vi "SalvarConfig.vi"(0 "caminho in":path, 1 "CanaisDinamicos":T2[](array[typedef]), 2 "CanaisEstaticos":string[][](array[string]), 3 "ConfigSistema":T1, 5 "error in":errorcluster) -> (14 "caminho out":path, 19 "error out":errorcluster)   [LabVIEW 2017]
uses:
  Typedefs/Tipo_DadosCanal.ctl
  Typedefs/Tipo_TipoSinalSimulado.ctl
  Typedefs/Tipo_ConfigSistema.ctl
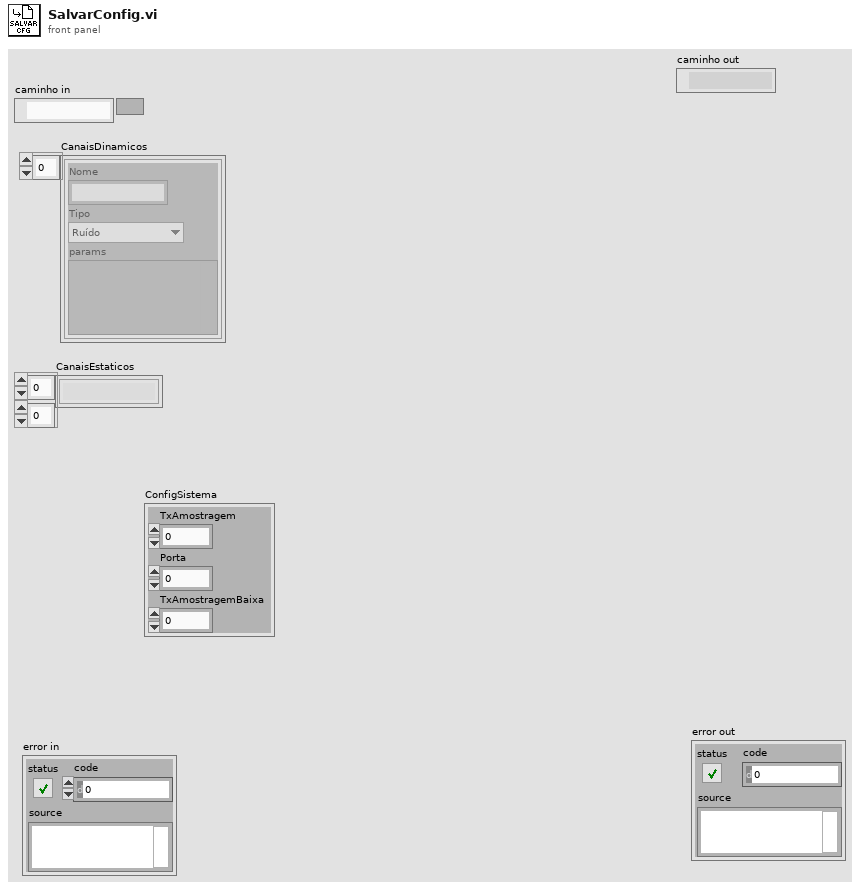
[diagram p1: front panel]
types:
  T1 = typedef "Tipo_ConfigSistema.ctl" = cluster{"TxAmostragem":dbl, "Porta":u16, "TxAmostragemBaixa":dbl}
  T2 = typedef "Tipo_DadosCanal.ctl" = cluster{"Nome":string, "Tipo":T3, "params":variant}
  T3 = typedef "Tipo_TipoSinalSimulado.ctl" = enum16{"Ruído", "Fasor", "Senóide", "Composto", "AM", "Proximidade", "Entreferro"}
  T4 = enum16{"open", "replace", "create", "open or create", "replace or create", "replace or create with confirmation"}
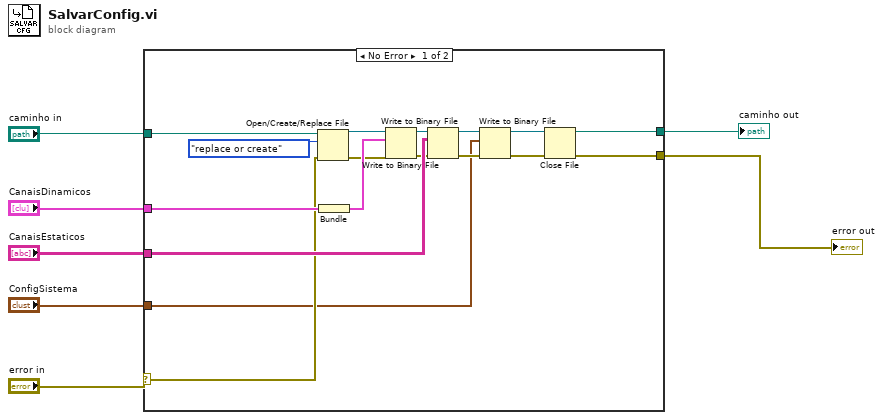
[diagram p0: block diagram]
diagram:
  n1 = case shown="No Error" "error in" {
    selector: "error in" -> [w12 w25]
    tunnel: "caminho in" -> [w24 w26]
    tunnel: "CanaisEstaticos" -> [w22 _]
    tunnel: "CanaisDinamicos" -> [w18 _]
    tunnel: [w17 w25] -> w4
    tunnel: [w13 w26] -> w3
    tunnel: "ConfigSistema" -> [w8 _]
    frame No Error {
      n2 = Open/Create/Replace File(file path (use dialog)=w24, error in=w12, operation (0:open)=T4."replace or create") -> (refnum out=w16:refnum<file>, error out=w15:errorcluster)  [unwired: 3 in, 1 out]
      n3 = Bundle("CanaisDinamicos"=w18) -> (w19:cluster{"CanaisDinamicos":T2[]})  [unwired: 1 in]
      n4 = Write to Binary File(file (use dialog)=w16, data=w19, error in=w15) -> (refnum out=w20:refnum<file>, error out=w21:errorcluster)  [unwired: 3 in, 1 out]
      n5 = Write to Binary File(file (use dialog)=w20, data=w22, error in=w21) -> (refnum out=w10:refnum<file>, error out=w23:errorcluster)  [unwired: 3 in, 1 out]
      n6 = Write to Binary File(file (use dialog)=w10, data=w8, error in=w23) -> (refnum out=w9:refnum<file>, error out=w11:errorcluster)  [unwired: 3 in, 1 out]
      n7 = Close File(refnum=w9, error in=w11) -> (path=w13:path, error out=w17:errorcluster)
    }
    frame Error {
    }
  }
  "error out" <- w4
  "caminho out" <- w3
